vi "LV SciSDK SPECTRUM START.vi"(0 "min":u32, 1 "max":u32=65535, 2 "limitmode":string(combo)="freerun", 3 "limit":u32, 5 "rebin":u32, 7 "Spectrum name":string, 9 "Board Handle In":T3, 11 "error in (no error)":errorcluster) -> (8 "Handle Out":T2, 10 "Board Handle Out":T1, 15 "error out":errorcluster)   [LabVIEW 2021, in "SciSDK_Labview.lvlib"]
doc: "You need this VI to execute 'start' spectrum component command"
uses:
  SciSDK_Labview.lvlib
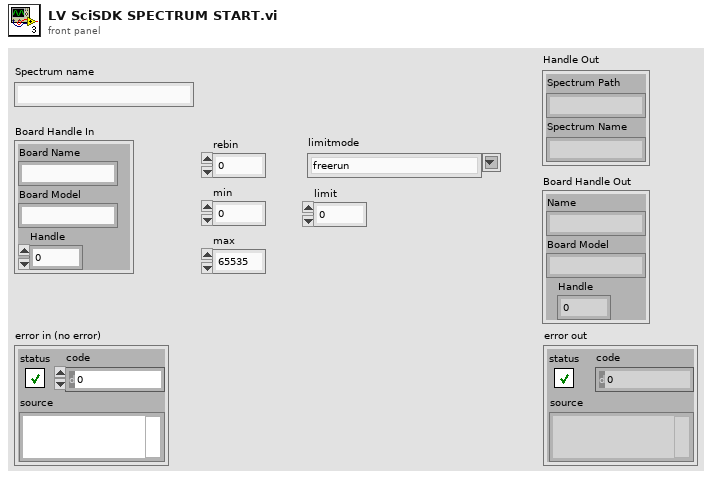
[diagram p1: front panel]
types:
  T1 = cluster{"Name":string, "Board Model":string, "Handle":u64}
  T2 = cluster{"Spectrum Path":string, "Spectrum Name":string}
  T3 = cluster{"Board Name":string, "Board Model":string, "Handle":u64}
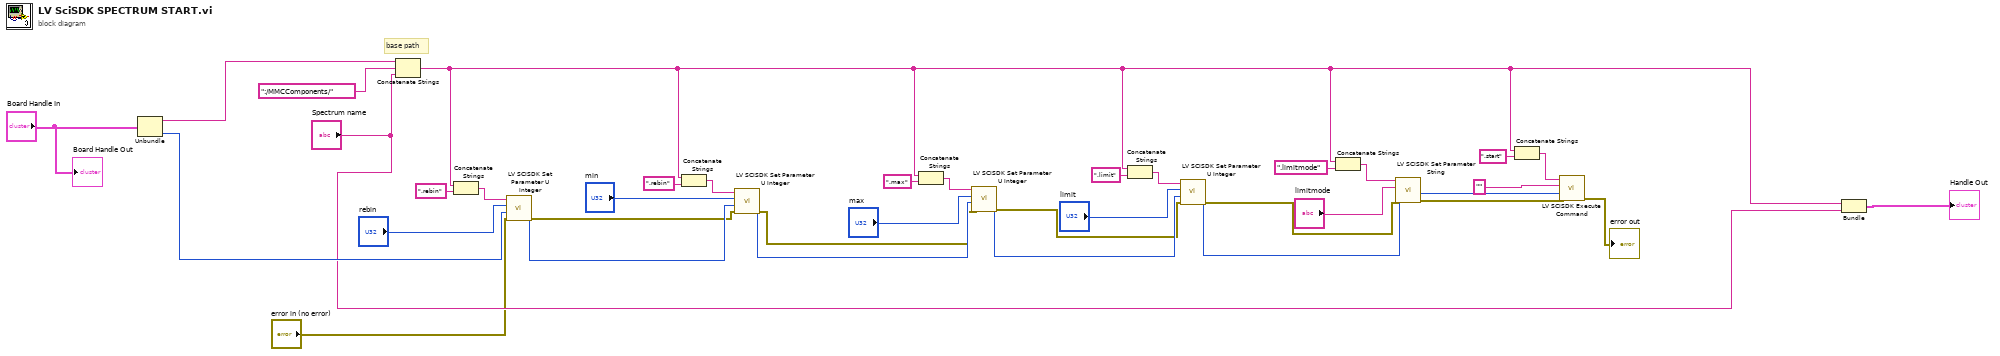
[diagram p0: block diagram]
diagram:
  # "base path"
  n1 = Unbundle("Board Handle In") -> ("Board Name"=w36:string, "Handle"=w32:u64)  [unwired: 1 out]
  n2 = Concatenate Strings(w36, ":/MMCComponents/" ("string"), "Spectrum name") -> (w9:string)
  n3 = Concatenate Strings(w9, ".rebin" ("string")) -> (w34:string)
  n4 = call "LV SCISDK Set Parameter U Integer.vi"("error in (no error)"="error in (no error)", "handle"=w32, "value"="rebin", "Path"=w34) -> ("error out"=w7:errorcluster, "handle out"=w25:u64)  [unwired: 5 in, 1 out]
  n5 = Concatenate Strings(w9, ".rebin" ("string")) -> (w30:string)
  n6 = call "LV SCISDK Set Parameter U Integer.vi"("error in (no error)"=w7, "handle"=w25, "value"="min", "Path"=w30) -> ("error out"=w6:errorcluster, "handle out"=w23:u64)  [unwired: 5 in, 1 out]
  n7 = Concatenate Strings(w9, ".max" ("string")) -> (w28:string)
  n8 = call "LV SCISDK Set Parameter U Integer.vi"("error in (no error)"=w6, "handle"=w23, "value"="max", "Path"=w28) -> ("error out"=w5:errorcluster, "handle out"=w21:u64)  [unwired: 5 in, 1 out]
  n9 = Concatenate Strings(w9, ".limit" ("string")) -> (w26:string)
  n10 = call "LV SCISDK Set Parameter U Integer.vi"("error in (no error)"=w5, "handle"=w21, "value"="limit", "Path"=w26) -> ("error out"=w4:errorcluster, "handle out"=w19:u64)  [unwired: 5 in, 1 out]
  n11 = Concatenate Strings(w9, ".limitmode" ("string")) -> (w16:string)
  n12 = call "LV SCISDK Set Parameter String.vi"("error in (no error)"=w4, "handle"=w19, "value"="limitmode", "Path"=w16) -> ("error out"=w3:errorcluster, "handle out"=w13:u64)  [unwired: 5 in, 1 out]
  n13 = Concatenate Strings(w9, ".start" ("string")) -> (w10:string)
  n14 = call "LV SCISDK Execute Command.vi"("error in (no error)"=w3, "handle"=w13, "value"="", "Path"=w10) -> ("error out"=→"error out":errorcluster)  [unwired: 5 in, 2 out]
  n15 = Bundle(w9, "Spectrum name"="Spectrum name") -> (→"Handle Out":cluster{string, "Spectrum name":string})  [unwired: 1 in]
  "Board Handle Out" <- "Board Handle In"
